vi "subStage_GetMinimumMovingDistance.vi"(8 "error in (no error)":errorcluster, 11 "XY Scan List":string[][](table)=[["1", "09/02 10:54:10", "1.4239", "1.7939", "Image", "green"], ["2", "09/02 10:54:22", "-0.5433", "-2.0517", "Image", "blue"], ["3", "09/02 10:54:29", "-1.9299", "-0.3478", "Image", "white"], ["4", "09/02 10:54:35", "1.8522", "-0.5608", "Image", "yellow"], ["5", "09/02 10:54:44", "2.5699", "-2.7322", "Image", "cyan"]]) -> (0 "error out":errorcluster, 3 "XY Scan List (reorder)":string[][](table)=[["", " ", "", ""], ["", " ", "", ""], ["", " ", "", ""], ["", " ", "", ""], ["", " ", "", ""]])   [LabVIEW 2015]
panel:
  out "XY Scan List deleted":string[][](table)
  out "Destination Point row index":i32=2
  out "Minimum distance":dbl=4.82593477
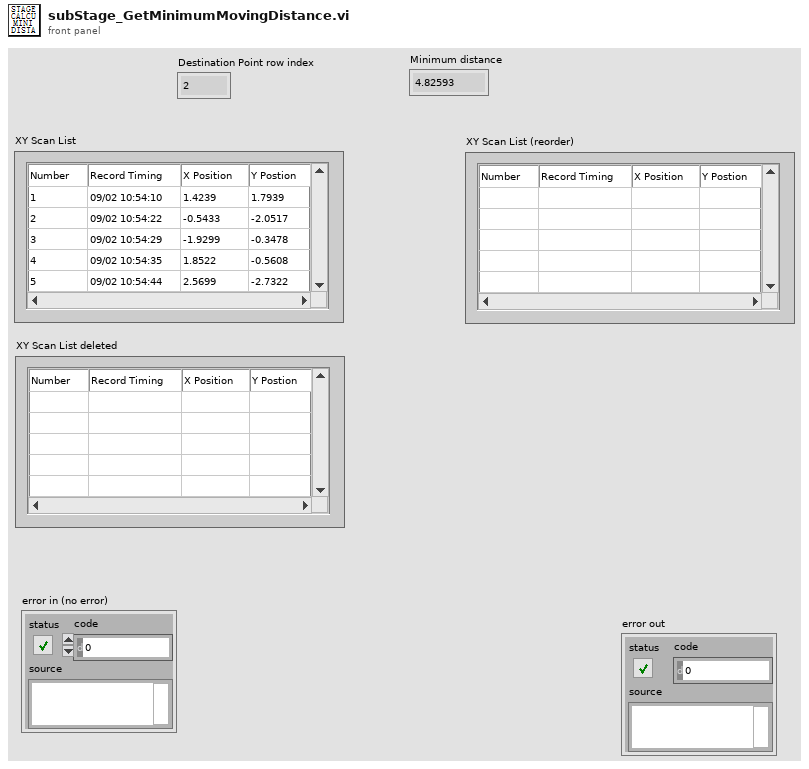
[diagram p1: front panel]
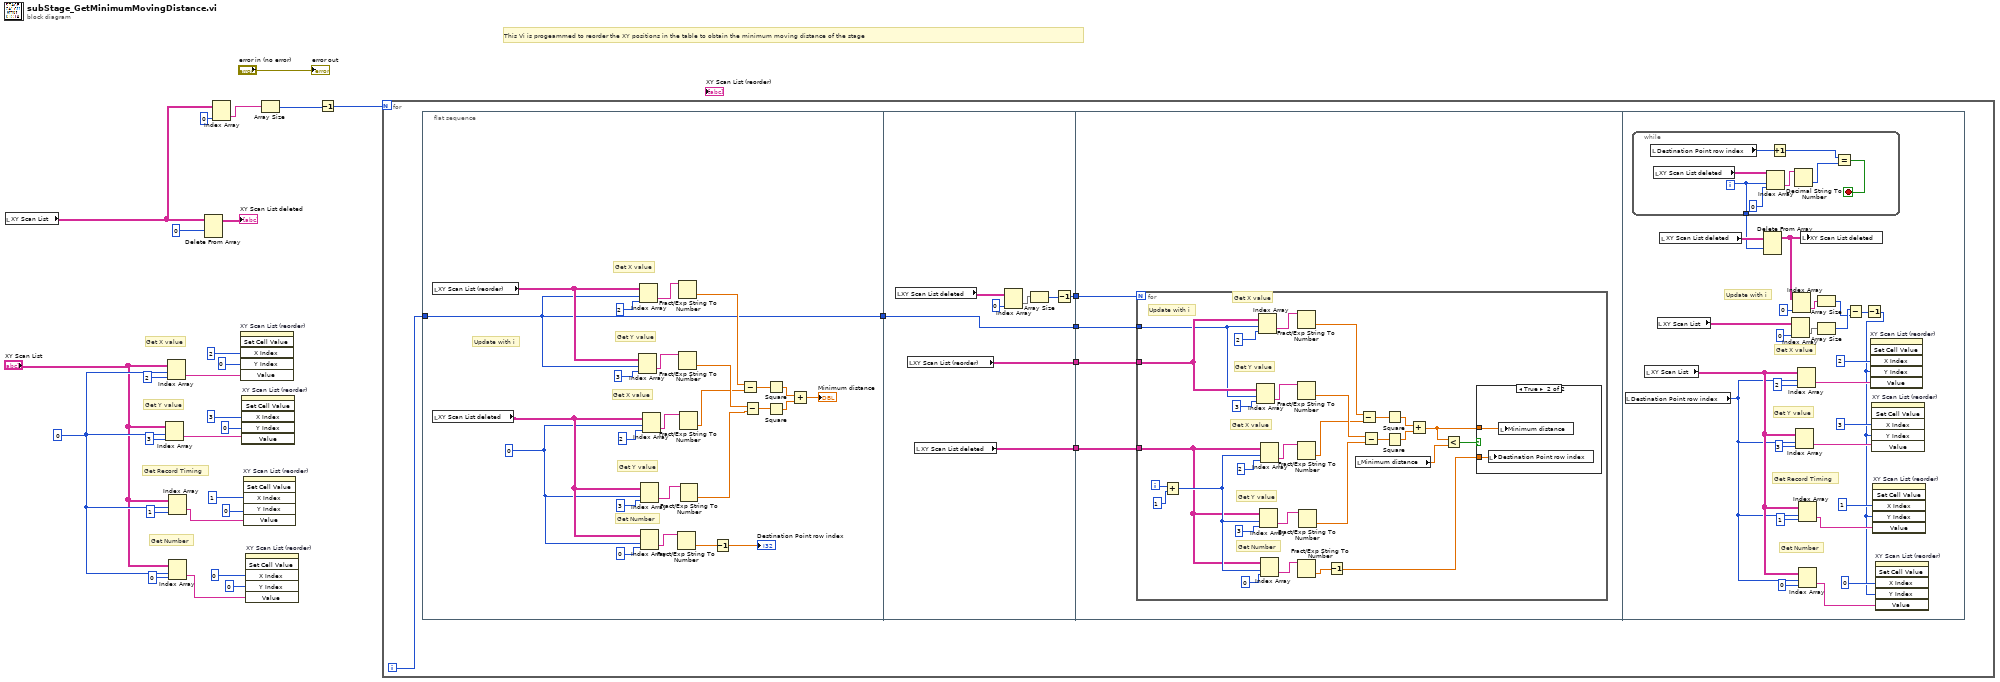
[diagram p0: block diagram]
diagram:
  w10 = 0
  # "This Vi is progeammed to reorder the XY positions in the table to obtain the minimum moving distance of the stage"
  # "Get Number"
  # "Get Record Timing"
  # "Get Y value"
  # "Get X value"
  n1 = local read "XY Scan List"() -> (w7:string[][])
  n2 = Index Array(array="XY Scan List", index (row)=w10, index (col)=3 ("disabled index (col)")) -> (element=w23:string)
  n3 = Index Array(array="XY Scan List", index (row)=w10, index (col)=2 ("disabled index (col)")) -> (element=w25:string)
  n4 = Index Array(array="XY Scan List", index (row)=w10, index (col)=1 ("disabled index (col)")) -> (element=w17:string)
  n5 = Index Array(array="XY Scan List", index (row)=w10, index (col)=0 ("disabled index (col)")) -> (element=w13:string)
  n6 = Delete From Array(array=w7, index (row)=0) -> (array with subset deleted=→"XY Scan List deleted":string[][])  [unwired: 2 in, 1 out]
  n7 = Index Array(array=w7, index (col)=0 ("disabled index (col)")) -> (element=w5:string[])  [unwired: 1 in]
  n8 = invoke on="XY Scan List (reorder)" class="Tbl (strict)" method="Set Cell Value"("X Index"=2, "Y Index"=0, "Value"=w25) -> ()  [unwired: 3 in, 6 out]
  n9 = invoke on="XY Scan List (reorder)" class="Tbl (strict)" method="Set Cell Value"("X Index"=3, "Y Index"=0, "Value"=w23) -> ()  [unwired: 3 in, 6 out]
  n10 = invoke on="XY Scan List (reorder)" class="Tbl (strict)" method="Set Cell Value"("X Index"=1, "Y Index"=0 ("X Index"), "Value"=w17) -> ()  [unwired: 3 in, 6 out]
  n11 = invoke on="XY Scan List (reorder)" class="Tbl (strict)" method="Set Cell Value"("X Index"=0, "Y Index"=0 ("X Index"), "Value"=w13) -> ()  [unwired: 3 in, 6 out]
  n12 = Array Size(array=w5) -> (size(s)=w4:i32)
  n13 = Decrement(x=w4) -> (x-1=w3:i32)
  n14 = for {
    N: w3 -> [_]
    i -> [w29]
    n15 = flat-sequence {
      tunnel: w29 -> [w33]
      tunnel: [w33] -> w27
      tunnel: [w62] -> w32
      tunnel: [w60] -> w31
      tunnel: [w58] -> w30
      tunnel: [w59] -> w28
      tunnel: w27 -> [w59]
      tunnel: w32 -> [w69]
      tunnel: w31 -> [w67]
      tunnel: w30 -> [w68]
      tunnel: w28 -> [w66]
      frame #0 {
        w36 = 0
        # "Get Number"
        # "Update with i"
        # "Get Y value"
        # "Get X value"
        # "Get Y value"
        # "Get X value"
        n16 = local read "XY Scan List (reorder)"() -> (w40:string[][])
        n17 = local read "XY Scan List deleted"() -> (w39:string[][])
        n18 = Index Array(array=w40, index (row)=w33, index (col)=3 ("disabled index (col)")) -> (element=w46:string)
        n19 = Index Array(array=w40, index (row)=w33, index (col)=2 ("disabled index (col)")) -> (element=w45:string)
        n20 = Index Array(array=w39, index (row)=w36, index (col)=3 ("disabled index (col)")) -> (element=w48:string)
        n21 = Index Array(array=w39, index (row)=w36, index (col)=0 ("disabled index (col)")) -> (element=w38:string)
        n22 = Index Array(array=w39, index (row)=w36, index (col)=2 ("disabled index (col)")) -> (element=w47:string)
        n23 = Fract/Exp String To Number(string=w38) -> (number=w35:dbl)  [unwired: 3 in, 1 out]
        n24 = Fract/Exp String To Number(string=w45) -> (number=w49:dbl)  [unwired: 3 in, 1 out]
        n25 = Fract/Exp String To Number(string=w46) -> (number=w51:dbl)  [unwired: 3 in, 1 out]
        n26 = Fract/Exp String To Number(string=w47) -> (number=w50:dbl)  [unwired: 3 in, 1 out]
        n27 = Fract/Exp String To Number(string=w48) -> (number=w52:dbl)  [unwired: 3 in, 1 out]
        n28 = Decrement(x=w35) -> (x-1=→"Destination Point row index":dbl)
        n29 = Subtract(x=w49, y=w50) -> (x-y=w53:dbl)
        n30 = Subtract(x=w51, y=w52) -> (x-y=w54:dbl)
        n31 = Square(x=w53) -> (x^2=w56:dbl)
        n32 = Square(x=w54) -> (x^2=w55:dbl)
        n33 = Add(x=w56, y=w55) -> (x+y=→"Minimum distance":dbl)
      }
      frame #1 {
        n34 = local read "XY Scan List deleted"() -> (w63:string[][])
        n35 = local read "XY Scan List (reorder)"() -> (w58:string[][])
        n36 = local read "XY Scan List deleted"() -> (w62:string[][])
        n37 = Index Array(array=w63, index (col)=0 ("disabled index (col)")) -> (element=w65:string[])  [unwired: 1 in]
        n38 = Array Size(array=w65) -> (size(s)=w61:i32)
        n39 = Decrement(x=w61) -> (x-1=w60:i32)
      }
      frame #2 {
        n40 = for {
          N: w67 -> [_]
          tunnel: w69 -> [w75]
          tunnel: w68 -> [w77]
          tunnel: w66 -> [w70]
          i -> [w83]
          # "Get Number"
          # "Update with i"
          # "Get Y value"
          # "Get X value"
          # "Get Y value"
          # "Get X value"
          n41 = Add(x=w83, y=1) -> (x+y=w76:i32)
          n42 = Index Array(array=w77, index (row)=w70, index (col)=3 ("disabled index (col)")) -> (element=w88:string)
          n43 = Index Array(array=w77, index (row)=w70, index (col)=2 ("disabled index (col)")) -> (element=w87:string)
          n44 = Index Array(array=w75, index (row)=w76, index (col)=3 ("disabled index (col)")) -> (element=w90:string)
          n45 = Index Array(array=w75, index (row)=w76, index (col)=0 ("disabled index (col)")) -> (element=w73:string)
          n46 = Index Array(array=w75, index (row)=w76, index (col)=2 ("disabled index (col)")) -> (element=w89:string)
          n47 = Fract/Exp String To Number(string=w87) -> (number=w91:dbl)  [unwired: 3 in, 1 out]
          n48 = Fract/Exp String To Number(string=w88) -> (number=w93:dbl)  [unwired: 3 in, 1 out]
          n49 = Fract/Exp String To Number(string=w89) -> (number=w92:dbl)  [unwired: 3 in, 1 out]
          n50 = Fract/Exp String To Number(string=w73) -> (number=w72:dbl)  [unwired: 3 in, 1 out]
          n51 = Fract/Exp String To Number(string=w90) -> (number=w94:dbl)  [unwired: 3 in, 1 out]
          n52 = Decrement(x=w72) -> (x-1=w71:dbl)
          n53 = local read "Minimum distance"() -> (w81:dbl)
          n54 = Subtract(x=w91, y=w92) -> (x-y=w95:dbl)
          n55 = Subtract(x=w93, y=w94) -> (x-y=w96:dbl)
          n56 = Square(x=w95) -> (x^2=w98:dbl)
          n57 = Square(x=w96) -> (x^2=w97:dbl)
          n58 = Add(x=w98, y=w97) -> (x+y=w78:dbl)
          n59 = Less?(x=w78, y=w81) -> (x < y?=w80:bool)
          n60 = case shown="True" w80 {
            tunnel: w78 -> [_ w100]
            tunnel: w71 -> [_ w99]
            frame False {
            }
            frame True {
              n61 = local write "Destination Point row index"(w99) -> ()
              n62 = local write "Minimum distance"(w100) -> ()
            }
          }
        }
      }
      frame #3 {
        # "Update with i"
        # "Get Number"
        # "Get Record Timing"
        # "Get Y value"
        # "Get X value"
        n63 = local read "Destination Point row index"() -> (w113:i32)
        n64 = while {
          tunnel: [w127] -> w101
          i -> [w127]
          stop <- w128 stop-if-true
          n65 = local read "Destination Point row index"() -> (w134:i32)
          n66 = local read "XY Scan List deleted"() -> (w133:string[][])
          n67 = Index Array(array=w133, index (row)=w127, index (col)=0 ("disabled index (col)")) -> (element=w131:string)
          n68 = Increment(x=w134) -> (x+1=w130:i32)
          n69 = Decimal String To Number(string=w131) -> (number=w129:i32)  [unwired: 2 in, 1 out]
          n70 = Equal?(x=w130, y=w129) -> (x = y?=w128:bool)
        }
        n71 = local read "XY Scan List"() -> (w114:string[][])
        n72 = local read "XY Scan List"() -> (w107:string[][])
        n73 = local read "XY Scan List deleted"() -> (w104:string[][])
        n74 = Delete From Array(array=w104, index (row)=w101) -> (array with subset deleted=w110:string[][])  [unwired: 2 in, 1 out]
        n75 = Index Array(array=w107, index (col)=0 ("disabled index (col)")) -> (element=w108:string[])  [unwired: 1 in]
        n76 = Index Array(array=w110, index (col)=0 ("disabled index (col)")) -> (element=w112:string[])  [unwired: 1 in]
        n77 = Index Array(array=w114, index (row)=w113, index (col)=3 ("disabled index (col)")) -> (element=w117:string)
        n78 = Index Array(array=w114, index (row)=w113, index (col)=2 ("disabled index (col)")) -> (element=w116:string)
        n79 = Index Array(array=w114, index (row)=w113, index (col)=1 ("disabled index (col)")) -> (element=w121:string)
        n80 = Index Array(array=w114, index (row)=w113, index (col)=0 ("disabled index (col)")) -> (element=w125:string)
        n81 = local write "XY Scan List deleted"(w110) -> ()
        n82 = Array Size(array=w112) -> (size(s)=w105:i32)
        n83 = Array Size(array=w108) -> (size(s)=w106:i32)
        n84 = Subtract(x=w106, y=w105) -> (x-y=w103:i32)
        n85 = Decrement(x=w103) -> (x-1=w102:i32)
        n86 = invoke on="XY Scan List (reorder)" class="Tbl (strict)" method="Set Cell Value"("X Index"=2, "Y Index"=w102, "Value"=w116) -> ()  [unwired: 3 in, 6 out]
        n87 = invoke on="XY Scan List (reorder)" class="Tbl (strict)" method="Set Cell Value"("X Index"=3, "Y Index"=w102, "Value"=w117) -> ()  [unwired: 3 in, 6 out]
        n88 = invoke on="XY Scan List (reorder)" class="Tbl (strict)" method="Set Cell Value"("X Index"=1, "Y Index"=w102, "Value"=w121) -> ()  [unwired: 3 in, 6 out]
        n89 = invoke on="XY Scan List (reorder)" class="Tbl (strict)" method="Set Cell Value"("X Index"=0, "Y Index"=w102, "Value"=w125) -> ()  [unwired: 3 in, 6 out]
      }
    }
  }
  "error out" <- "error in (no error)"
